vi "Get Keywords.vi"(8 "error in (no error)":errorcluster, 11 "scripts manager in":refnum<class "scripts manager.lvclass">) -> (0 "error out":errorcluster, 2 "Keywords":string[](array[string]), 3 "scripts manager out":refnum<class "scripts manager.lvclass">)   [LabVIEW 2019, in "LSL.lvlib" / "scripts manager.lvclass"]
uses:
  scripts manager.lvclass
  scripts manager.lvclass/scripts manager.ctl
  functions/functionsbase/functionbase.lvclass
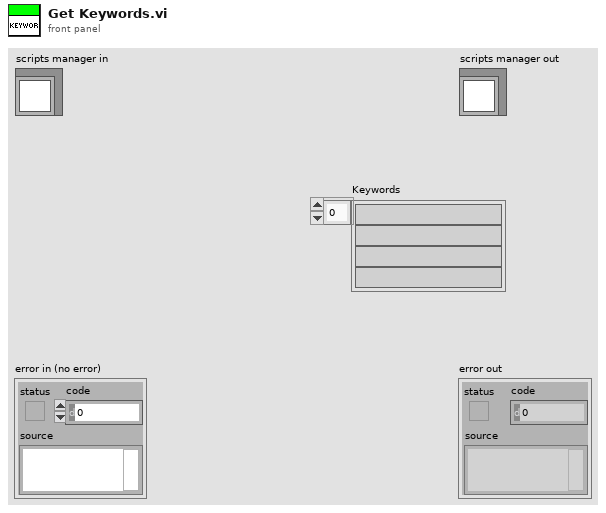
[diagram p1: front panel]
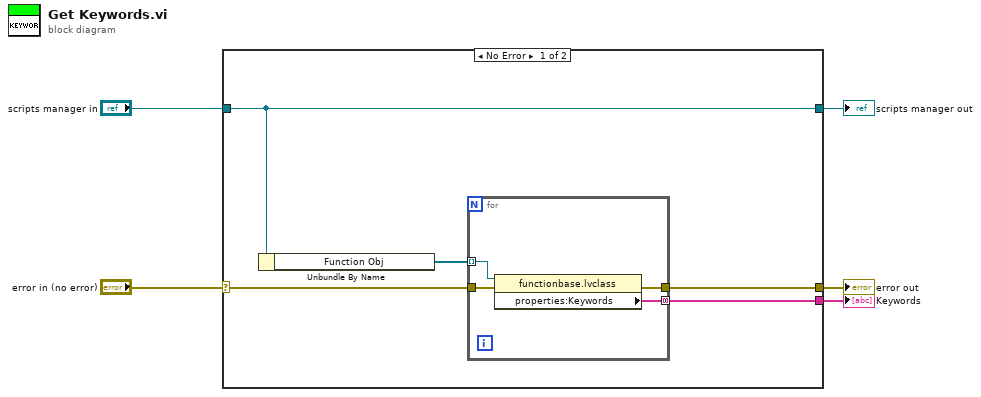
[diagram p0: block diagram]
diagram:
  n1 = case shown="No Error" "error in (no error)" {
    selector: "error in (no error)" -> [w8 w16]
    tunnel: [w7 w16] -> w4
    tunnel: [w10 w15] -> w2
    tunnel: "scripts manager in" -> [w10 w15]
    tunnel: [w6 _] -> w1
    frame No Error {
      n2 = Unbundle By Name(w10) -> ("Function Obj"=w9:refnum<class "functionbase.lvclass">[])
      n3 = for {
        tunnel: w9 -> [w12] mode=indexing
        tunnel: w8 -> [w14]
        tunnel: [w13] -> w7
        tunnel: [w11] -> w6 mode=concatenating
        n4 = property class="functionbase.lvclass"(reference=w12, error in=w14) -> (error out=w13:errorcluster, "properties:Keywords"=w11:string[])  [unwired: 1 out]
      }
    }
    frame Error {
    }
  }
  "error out" <- w4
  "scripts manager out" <- w2
  "Keywords" <- w1
